vi "HAL camera start acquire.vi"(1 "error in":errorcluster) -> (0 "error out":errorcluster)   [LabVIEW 2011]
doc: "Starts an iXon acquisition (if not already running)"
uses:
  HAL Camera specifications globals.vi
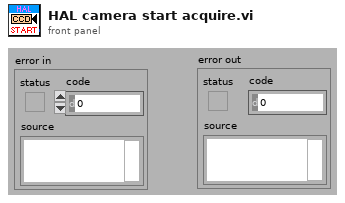
[diagram p1: front panel]
types:
  T1 = cluster{"width":u32, "height":u32, "datatype":u32}
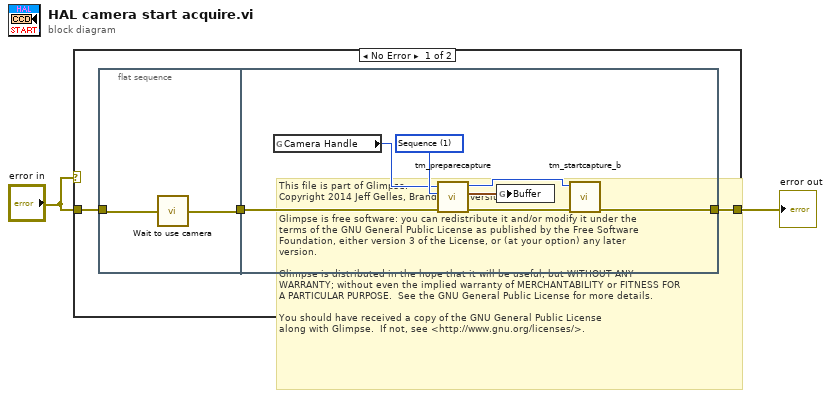
[diagram p0: block diagram]
diagram:
  # "This file is part of Glimpse. \nCopyright 2014 Jeff Gelles, Brandeis University.    \n\nGlimpse is free software: you can redistribute it and/or modify it under the \nterms of the GNU General Public License as published by the Free Software \nFoundation, either version 3 of the License, or (at your option) any later \nversion.\n\nGlimpse is distributed in the hope that it will be useful, but WITHOUT ANY \nWARRANTY; without even the implied warranty of MERCHANTABILITY or FITNESS FOR \nA PARTICULAR PURPOSE.  See the GNU General Public License for more details.\n\nYou should have received a copy of the GNU General Public License\nalong with Glimpse.  If not, see <http://www.gnu.org/licenses/>."
  n1 = case shown="No Error" "error in" {
    tunnel: "error in" -> [w5 w15]
    tunnel: [w4 w15] -> w2
    frame No Error {
      n2 = flat-sequence {
        tunnel: w5 -> [w6]
        tunnel: [w7] -> w3
        tunnel: [w14] -> w4
        tunnel: w3 -> [w9]
        frame #0 {
          n3 = call "Wait to use camera.vi"("error in"=w6) -> ("error out"=w7:errorcluster)
        }
        frame #1 {
          w13 = 1 items=["Snap", "Sequence"] ("Capture mode")
          n4 = global read "HAL Camera specifications globals.vi" "Camera Handle"() -> (w11:u32)
          n5 = call <userlib>:"tm_preparecapture.vi"("error in (no error)"=w9, "Capture mode"=w13, "Handle in"=w11) -> ("error out"=w8:errorcluster, "Buffer"=w12:T1, "Handle out"=w10:u32)  [unwired: 5 in, 1 out]
          n6 = global write "HAL Camera specifications globals.vi" "Buffer"(w12) -> ()
          n7 = call <userlib>:"tm_startcapture_b.vi"("error in (no error)"=w8, "Handle in"=w10) -> ("error out"=w14:errorcluster)  [unwired: 8 in, 1 out]
        }
      }
    }
    frame Error {
    }
  }
  "error out" <- w2
